vi "AMGenViTest.vi"() -> ()   [LabVIEW 2018]
uses:
  <vilib>/measure/NI_MABase.lvlib
panel:
  out "AMOutput":waveform(dbl)[](graph)
  out "ModulationWave":waveform(dbl)[](graph)
  out "CarrierWave":waveform(dbl)[](graph)
  out "FFTWave":cluster{"f0":dbl, "df":dbl, "magnitude":dbl[]}[](graph)
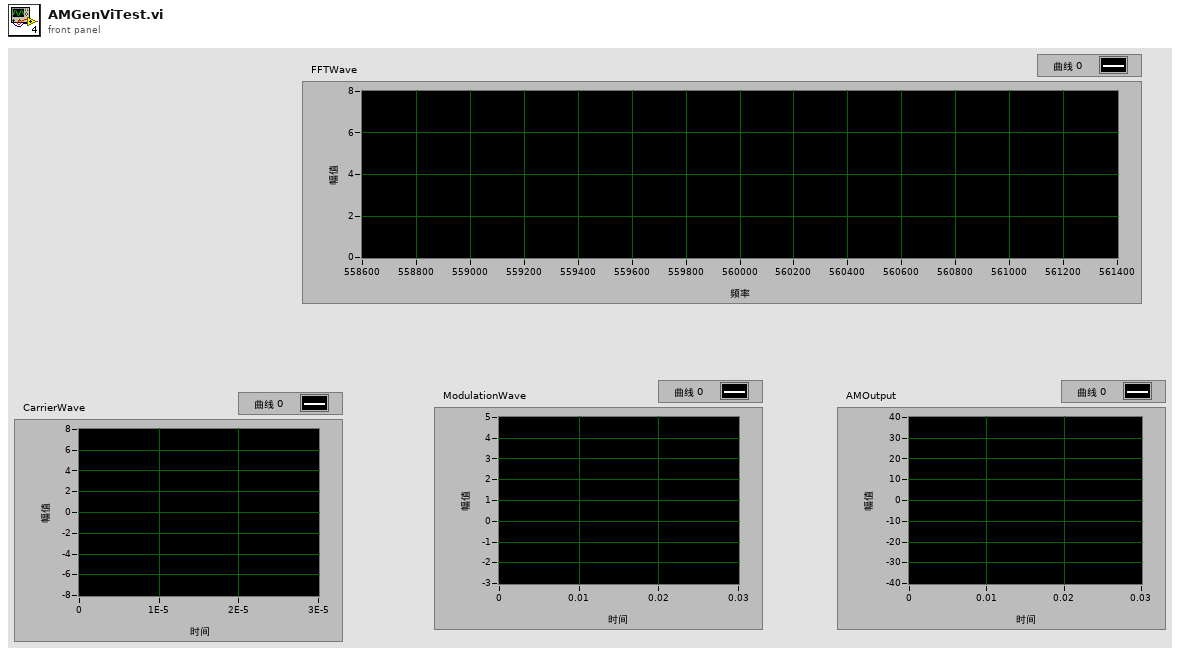
[diagram p1: front panel]
types:
  T1 = cluster{"Array of Waveform":waveform(dbl)[], waveform(dbl)[], waveform(dbl)[]}
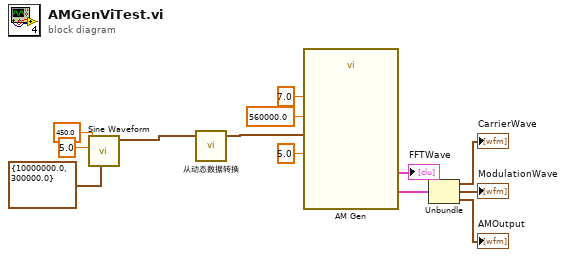
[diagram p0: block diagram]
diagram:
  n1 = call <vilib>:"Sine Waveform.vi"("sampling info"=cluster{"Fs":dbl, "#s":dbl} {"Fs"=10000000.0, "#s"=300000.0}, "amplitude"=5.0, "frequency"=450.0) -> ("signal out"=w7:waveform(dbl))  [unwired: 7 in, 1 out]
  n2 = call "从动态数据转换"("Dynamic Data Type"=w7) -> ("Array of Waveform"=w8:waveform(dbl)[])  [unwired: 3 in]
  n3 = call "AM Gen.vi"("MIDI Waveform"=w8, "ModulationAmp"=5.0, "CarrierFre"=560000.0, "CarrierAmp"=7.0) -> ("FFTWave"=→"FFTWave":cluster{"f0":dbl, "df":dbl, "magnitude":dbl[]}[], "输出簇"=w12:T1)  [unwired: 6 in]
  n4 = Unbundle(w12) -> ("Array of Waveform"=→"CarrierWave":waveform(dbl)[], →"ModulationWave":waveform(dbl)[], →"AMOutput":waveform(dbl)[])
